vi "Pre Launch Init.vi"(11 "IMAQ Display in":refnum<class "HIJ Vision Display.lvclass">) -> (0 "error out":errorcluster, 3 "IMAQ Display out":refnum<class "HIJ Vision Display.lvclass">)   [LabVIEW 2014, in "HIJ Vision Display.lvlib" / "HIJ Vision Display.lvclass"]
doc: "(<B>Filename</B>: Actor Framework.lvlib:Actor.lvclass:Pre Launch Init.vi)\n\nDefines behavior that occurs after the Launch Actor method is invoked but before the actor's Actor Core method begins running.\n\nThe Pre Launch Init method is guaranteed to finish before the Launch Actor method returns to its caller and before the actor itself receives any messages. Any references that the Pre Launch Init method obtains are guaranteed to have the same lifetime as the actor itself. Any errors that the Pre Launch Init method returns will abort the launch.\n\nBy default, this method does nothing. A descendant class may override it to define behavior."
uses:
  HIJ Vision Display.lvclass
  HIJ Vision Display.lvclass/HIJ Vision Display.ctl
  Shared Code/Viewable Actor/ViewableActor/ViewableActor.lvclass
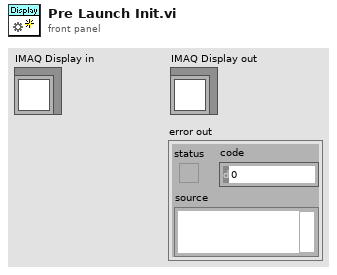
[diagram p1: front panel]
types:
  T1 = typedef "Image Type" = u32
  T2 = typedef "IMAQ Image.ctl" = refnum<image>
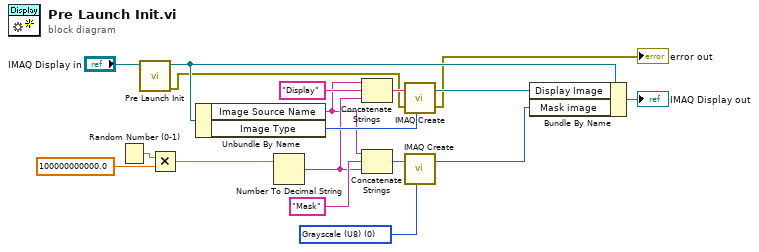
[diagram p0: block diagram]
diagram:
  w5 = T1 0 items=["Grayscale (U8)", "Grayscale (I16)", "Grayscale (SGL)", "Complex (CSG)", "RGB (U32)", "HSL (U32)", "RGB (U64)", "Grayscale (U16)"] ("Image Type")
  n1 = Random Number (0-1)() -> (number: 0 to 1=w12:dbl)
  n2 = call-parent "Pre Launch Init.vi"("ViewableActor in"="IMAQ Display in") -> ("error out"=w1:errorcluster, "ViewableActor out"=w14:refnum<class "HIJ Vision Display.lvclass">)  [unwired: 9 in]
  n3 = Multiply(x=w12, y=100000000000.0) -> (x*y=w10:dbl)
  n4 = Unbundle By Name(w14) -> ("Image Source Name"=w7:string, "Image Type"=w15:T1)
  n5 = Number To Decimal String(number=w10) -> (decimal integer string=w8:string)  [unwired: 1 in]
  n6 = Concatenate Strings(w7, "Display" ("string"), w8) -> (w17:string)
  n7 = Concatenate Strings(w7, "Mask" ("string"), w8) -> (w6:string)
  n8 = call "IMAQ Create"("Image Name"=w17, "Image Type"=w15, "error in (no error)"=w1) -> ("New Image"=w3:T2, "error out"=→"error out":errorcluster)  [unwired: 2 in]
  n9 = call "IMAQ Create"("Image Name"=w6, "Image Type"=w5) -> ("New Image"=w4:T2)  [unwired: 3 in, 1 out]
  n10 = Bundle By Name(cluster=w14, "Display Image"=w3, "Mask image"=w4) -> (→"IMAQ Display out":refnum<class "HIJ Vision Display.lvclass">)
